vi "Import_Old.vi"(1 "Input Sequence":T1(array[cluster])) -> (0 "Output Sequence":T1(array[cluster]))   [LabVIEW 2011]
doc: "This VI makes changes to the sequence to fix errors with files authored by old versions of the Growth Sequence Editor."
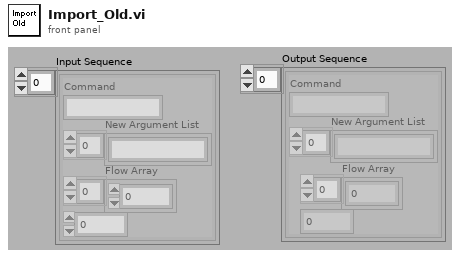
[diagram p1: front panel]
types:
  T1 = cluster{"Command":string, "New Argument List":string[], "Flow Array":dbl[], dbl}[]
  T2 = cluster{"Command":string, "New Argument List":string[], "Flow Array":dbl[], dbl}
  T3 = cluster{string, "New Argument List":string[], "Flow Array":dbl[], dbl}
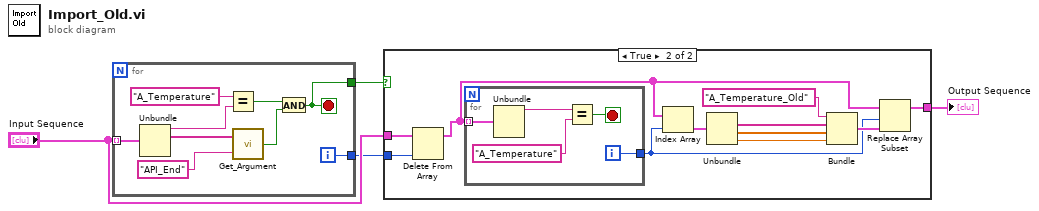
[diagram p0: block diagram]
diagram:
  n1 = for {
    tunnel: "Input Sequence" -> [w13] mode=indexing
    tunnel: [w6] -> w3
    tunnel: [w5] -> w2
    i -> [w6]
    stop <- w5 stop-if-true
    n2 = Unbundle(w13) -> ("Command"=w10:string, "New Argument List"=w12:string[])  [unwired: 2 out]
    n3 = Equal?(x="A_Temperature", y=w10) -> (x = y?=w8:bool)
    n4 = call "Get_Argument.vi"("Argument"="API_End", "Argument List"=w12) -> ("Enabled"=w7:bool)
    n5 = And(x=w8, y=w7) -> (x .and. y?=w5:bool)
  }
  n6 = case shown="True" w2 {
    tunnel: "Input Sequence" -> [w14 w24]
    tunnel: w3 -> [_ w25]
    tunnel: [w14 w16] -> w1
    frame False {
    }
    frame True {
      n7 = Delete From Array(array=w24, index=w25) -> (array with subset deleted=w17:T1)  [unwired: 1 in, 1 out]
      n8 = for {
        tunnel: w17 -> [w30] mode=indexing
        tunnel: [w26] -> w15
        i -> [w26]
        stop <- w27 stop-if-true
        n9 = Unbundle(w30) -> ("Command"=w29:string)  [unwired: 3 out]
        n10 = Equal?(x=w29, y="A_Temperature") -> (x = y?=w27:bool)
      }
      n11 = Index Array(array=w17, index=w15) -> (element=w23:T2)
      n12 = Unbundle(w23) -> ("New Argument List"=w20:string[], "Flow Array"=w21:dbl[], w22:dbl)  [unwired: 1 out]
      n13 = Bundle("A_Temperature_Old", "New Argument List"=w20, "Flow Array"=w21, w22) -> (w18:T3)  [unwired: 1 out]
      n14 = Replace Array Subset(array=w17, new element=w18, index=w15) -> (w16:T1)
    }
  }
  "Output Sequence" <- w1
